vi "StartSeparateServer.vi"(3 "Server":string) -> (0 "error out":errorcluster, 1 "Ref out":refnum<vi>)   [LabVIEW 2015]
doc: "Opens a VI Reference for a new server"
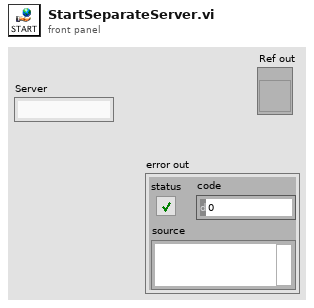
[diagram p1: front panel]
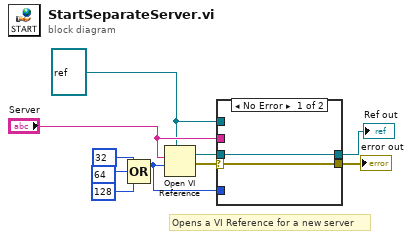
[diagram p0: block diagram]
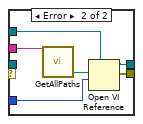
[diagram p2: hidden frame]
diagram:
  w2 = refnum<vi> refnum ("type specifier VI Refnum (for type only)")
  # "Opens a VI Reference for a new server"
  n1 = Compound Arithmetic op=OR(32, 64, 128) -> (w8:i32)
  n2 = Open VI Reference(type specifier VI Refnum (for type only)=w2, vi path="Server", options=w8) -> (vi reference=w6:refnum<vi>, error out=w7:errorcluster)  [unwired: 3 in]
  n3 = case shown="No Error" w7 {
    selector: w7 -> [w12 _]
    tunnel: w2 -> [_ w18]
    tunnel: w8 -> [_ w17]
    tunnel: [w11 w16] -> w1
    tunnel: [w12 w15] -> w9
    tunnel: w6 -> [w11 _]
    tunnel: "Server" -> [_ w14]
    frame No Error {
    }
    frame Error {
      n4 = call "GetAllPaths.vi"("LocalName"=w14) -> ("Hard Path"=w13:path)  [unwired: 2 out]
      n5 = Open VI Reference(type specifier VI Refnum (for type only)=w18, vi path=w13, options=w17) -> (vi reference=w16:refnum<vi>, error out=w15:errorcluster)  [unwired: 3 in]
    }
  }
  "error out" <- w9
  "Ref out" <- w1
